vi "SaveArrayTiff.vi"(5 "name":string="D:\\Data\\Mai\\2019-03-08\\images raw\\test", 6 "Target Folder":path, 8 "error in (no error)":errorcluster, 10 "output array":u16[][](array[numeric]), 11 "number":dbl format="%#_13g") -> (0 "error out":errorcluster)   [LabVIEW 2018, in "RW_Protocols.lvlib"]
uses:
  RW_Protocols.lvlib
  FileType.ctl
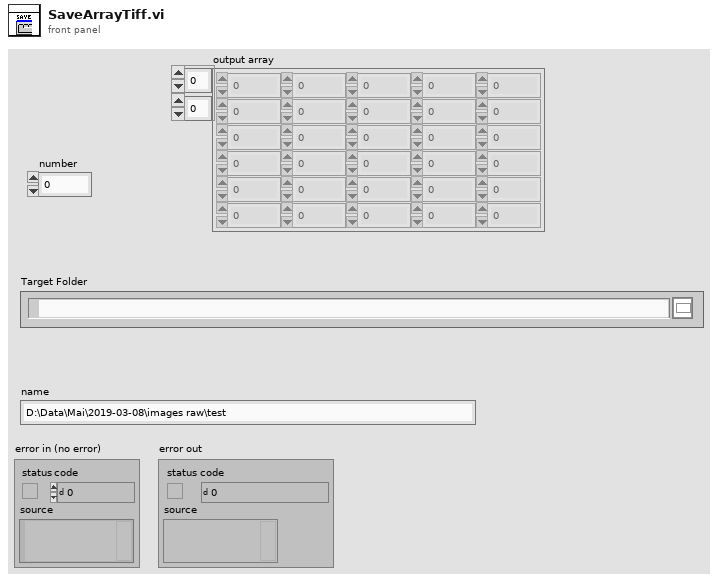
[diagram p1: front panel]
types:
  T1 = typedef "Image Type" = u32
  T2 = typedef "RW_Protocols.lvlib/FileType.ctl" = enum16{"png", "csv", "tiff", "dat", "bin", "txt"}
  T3 = typedef "IMAQ Image.ctl" = refnum<image>
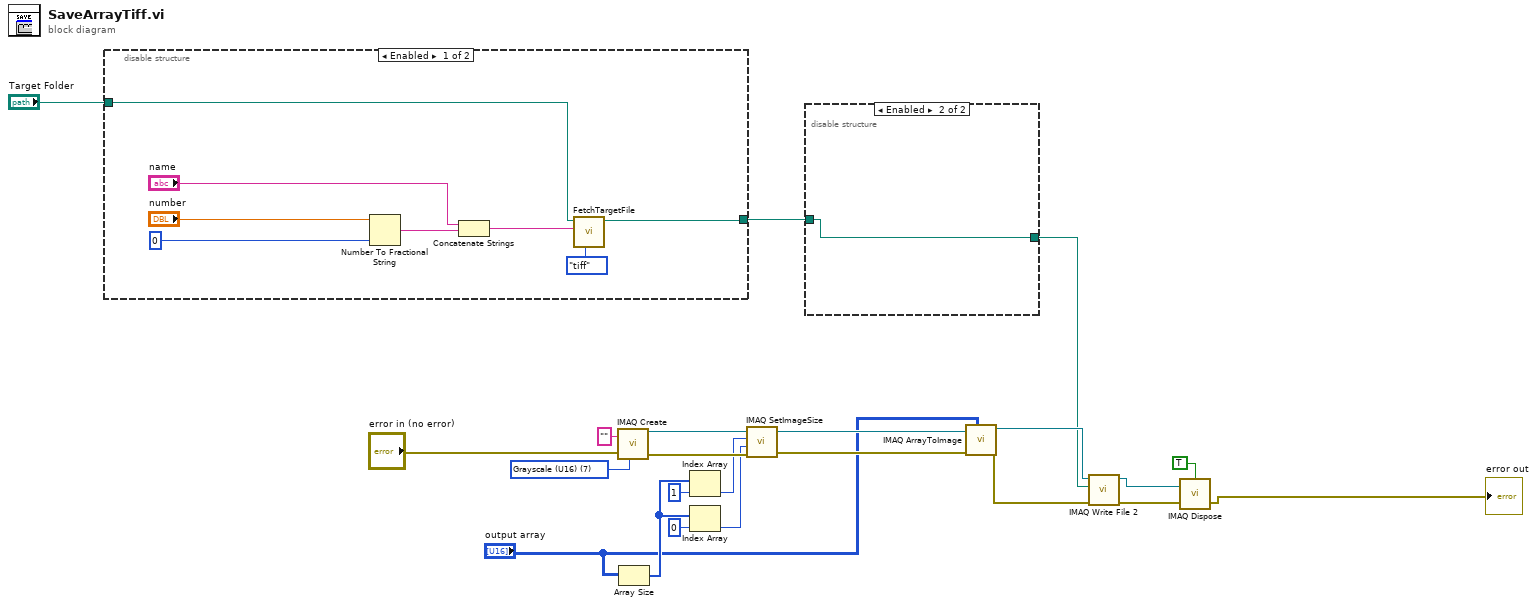
[diagram p0: block diagram]
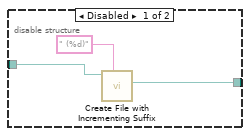
[diagram p2: hidden frame]
diagram:
  w21 = T1 7 items=["Grayscale (U8)", "Grayscale (I16)", "Grayscale (SGL)", "Complex (CSG)", "RGB (U32)", "HSL (U32)", "RGB (U64)", "Grayscale (U16)"] ("Image Type")
  n1 = disable-structure shown="Enabled" {
    disable-tunnel: "Target Folder" -> [w24 w31]
    disable-tunnel: [w25 w31] -> w2
    frame Enabled {
      n2 = Number To Fractional String(number="number", precision (6)=i16 0) -> (F-format string=w30:string)  [unwired: 2 in]
      n3 = Concatenate Strings("name", w30) -> (w26:string)
      n4 = call "FetchTargetFile.vi"("file type"=FileType."tiff", "FileName"=w26, "Target Folder"=w24) -> ("Full File Path"=w25:path)  [unwired: 7 in, 1 out]
    }
    frame Disabled {
    }
  }
  n5 = call "IMAQ Create"("Image Name"="", "Image Type"=w21, "error in (no error)"="error in (no error)") -> ("New Image"=w18:T3, "error out"=w20:errorcluster)  [unwired: 2 in]
  n6 = Array Size(array="output array") -> (size(s)=w14:i32[])
  n7 = Index Array(array=w14, index=1) -> (element=w12:i32)
  n8 = Index Array(array=w14, index=0) -> (element=w15:i32)
  n9 = call "IMAQ SetImageSize"("error in (no error)"=w20, "Y Resolution"=w15, "X Resolution"=w12, "Image"=w18) -> ("error out"=w19:errorcluster, "Image Out"=w17:T3)  [unwired: 1 in]
  n10 = disable-structure shown="Enabled" {
    disable-tunnel: w2 -> [w34 w35]
    disable-tunnel: [w33 w35] -> w1
    frame Disabled {
      n11 = call <vilib>:"Create File with Incrementing Suffix.vi"("format string (\" (%d)\")"=" (%d)" ("format string (\" (%d)\")"), "file path"=w34) -> ("actual path"=w33:path)  [unwired: 7 in, 2 out]
    }
    frame Enabled {
    }
  }
  n12 = call "IMAQ ArrayToImage"("Image Pixels (U16)"="output array", "error in (no error)"=w19, "Image"=w17) -> ("error out"=w9:errorcluster, "Image Out"=w8:T3)  [unwired: 7 in]
  n13 = call-poly "IMAQ Write File 2"("error in (no error)"=w9, "File Path"=w1, "Image"=w8) -> ("error out"=w7:errorcluster, "Image Out (duplicate)"=w6:T3)  [unwired: 7 in]
  n14 = call "IMAQ Dispose"("All Images? (No)"=TRUE, "Image"=w6, "error in (no error)"=w7) -> ("error out"=→"error out":errorcluster)  [unwired: 3 in]
